vi "Device Buffer.vi"(7 "States":T2=enum."Add", 8 "Error In":errorcluster, 11 "Device":T1) -> (0 "Error Out":errorcluster, 3 "Device Out":T1)   [LabVIEW 2012, in "OpenCLV x64.lvlib"]
doc: "Adds a device handle to a Labview buffer that can be used to clean-up devices later."
uses:
  OpenCLV x64.lvlib
  Controls/Device ID.ctl
  Buffer_states.ctl
  Error Checking/Add Error Functional Global.vi
panel:
  in  "Platform":u64
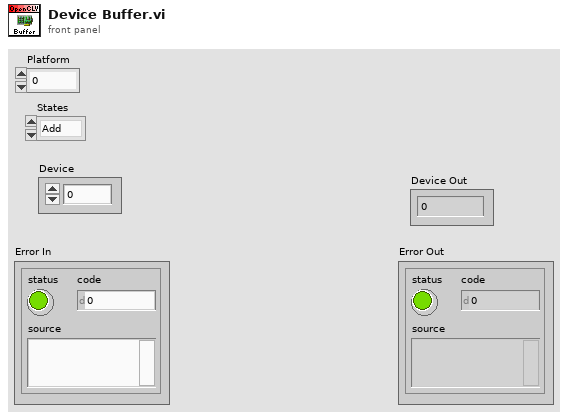
[diagram p1: front panel]
types:
  T1 = typedef "OpenCLV x64.lvlib/Device ID.ctl" = u64
  T2 = typedef "OpenCLV x64.lvlib/Buffer_states.ctl" = enum16{"Purge", "Remove", "Add"}
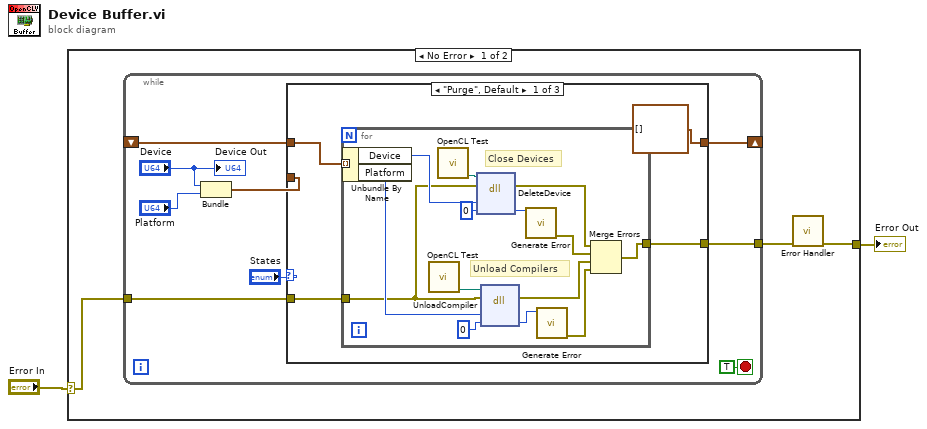
[diagram p0: block diagram]
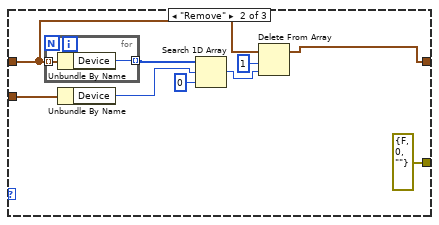
[diagram p2: hidden frame]
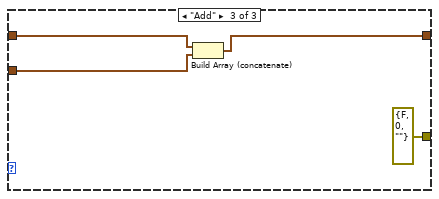
[diagram p3: hidden frame]
diagram:
  n1 = case shown="No Error" "Error In" {
    selector: "Error In" -> [w3 w49]
    tunnel: [w4 w49] -> w1
    frame No Error {
      n2 = while {
        shift-right: [w11] -> _
        shift-left: _ -> [w12]
        tunnel: [w10] -> w5
        tunnel: w3 -> [w6]
        stop <- TRUE stop-if-true
        n3 = Bundle("Device"="Device", "Platform"="Platform") -> (w8:cluster{"Device":T1, "Platform":u64})  [unwired: 1 in]
        n4 = case shown="\"Purge\", Default" "States" {
          tunnel: w8 -> [_ w36 w47]
          tunnel: w12 -> [w18 w38 w48]
          tunnel: [cluster{"Device":T1, "Platform":u64}[] [] w37 w46] -> w11
          tunnel: [w17 errorcluster {"status"=FALSE, "code"=0, "source"=""} ("error IO") errorcluster {"status"=FALSE, "code"=0, "source"=""} ("error IO")] -> w10
          tunnel: w6 -> [w15 _ _]
          frame "Purge", Default {
            n5 = for {
              tunnel: w18 -> [w31] mode=indexing
              tunnel: [w25] -> w17
              tunnel: w15 -> [w22]
              # "Unload Compilers"
              # "Close Devices"
              n6 = Unbundle By Name(w31) -> ("Device"=w30:T1, "Platform"=w29:u64)
              n7 = call "OpenCL Test.vi"() -> ("DLL To Use"=w23:path)  [unwired: 11 in]
              n8 = call "OpenCL Test.vi"() -> ("DLL To Use"=w24:path)  [unwired: 11 in]
              n9 = dll-call lib="C:/Users/bme-amcelroy-la/Desktop/OpenCLV/trunk/OpenCLV_x64_1.0/OpenCLV_x64.dll" fn="DeleteDevice"(path in=w24, error in=w22, "Device Handle"=w30, "Error"=0) -> (error out=w21:errorcluster, "Error"=w32:i32)  [unwired: 3 in, 1 out]
              n10 = dll-call lib="C:/Users/bme-amcelroy-la/Desktop/OpenCLV/trunk/OpenCLV_x64_1.0/OpenCLV_x64.dll" fn="UnloadCompiler"(path in=w23, error in=w22, "Device Handle"=w29, "Error"=0) -> (error out=w20:errorcluster, "Error"=w27:i32)  [unwired: 3 in, 1 out]
              n11 = call "Generate Error.vi"("Error"=w32) -> ("error out"=w26:errorcluster)  [unwired: 10 in]
              n12 = call "Generate Error.vi"("Error"=w27) -> ("error out"=w19:errorcluster)  [unwired: 10 in]
              n13 = Merge Errors(w21, w26, w20, w19) -> (w25:errorcluster)
            }
          }
          frame "Remove" {
            n14 = for {
              tunnel: w38 -> [w44] mode=indexing
              tunnel: [w43] -> w39 mode=indexing
              n15 = Unbundle By Name(w44) -> ("Device"=w43:T1)
            }
            n16 = Unbundle By Name(w36) -> ("Device"=w35:T1)
            n17 = Search 1D Array(1D array=w39, element=w35, start index (0)=0) -> (index of element=w40:i32)
            n18 = Delete From Array(array=w38, length=1, index=w40) -> (array with subset deleted=w37:cluster{"Device":T1, "Platform":u64}[])  [unwired: 1 out]
          }
          frame "Add" {
            n19 = Build Array (concatenate)(w48, w47) -> (w46:cluster{"Device":T1, "Platform":u64}[])
          }
        }
        "Device Out" <- "Device"
      }
      n20 = call-poly "Error Handler.vi"("Error In"=w5) -> ("Error Out"=w4:errorcluster)  [unwired: 10 in]
    }
    frame Error {
    }
  }
  "Error Out" <- w1
